vi "Start FFMpeg Process.vi"(8 "error in (no error)":errorcluster, 10 "Arguments":string, 11 "FFMPEG exe":path) -> (0 "error out":errorcluster, 3 "FFMpegProcess":T1)   [LabVIEW 2025]
uses:
  controls/FFMpegRef.ctl
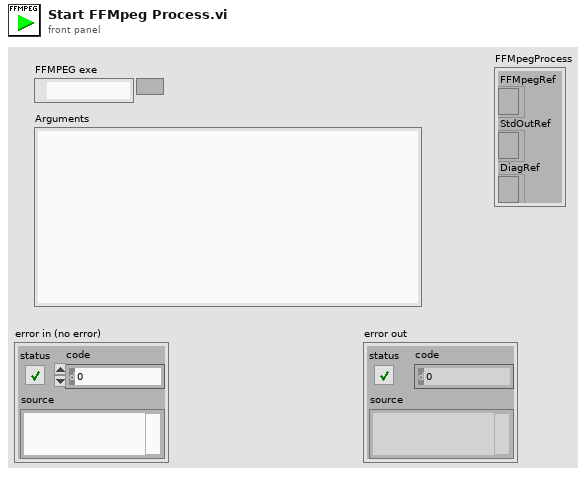
[diagram p1: front panel]
types:
  T1 = typedef "FFMpegRef.ctl" = cluster{"FFMpegRef":refnum<k24>, "StdOutRef":refnum<k24>, "DiagRef":refnum<k24>}
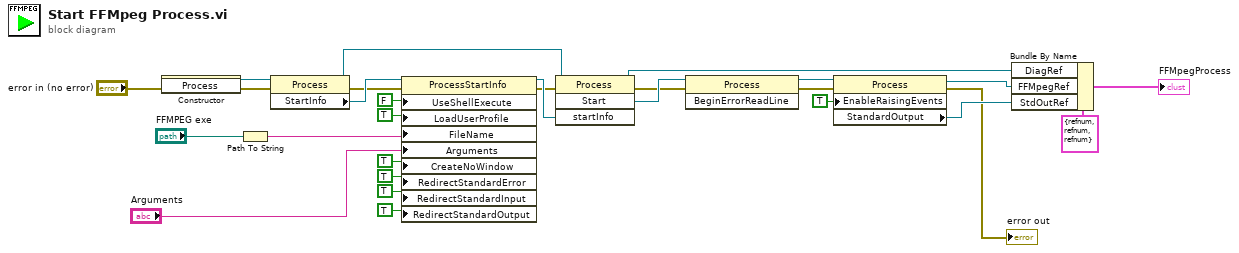
[diagram p0: block diagram]
diagram:
  n1 = constructor class="Process"(error in="error in (no error)") -> (reference out=w20:refnum<k24>, error out=w3:errorcluster)  [unwired: 2 in, 1 out]
  n2 = Path To String(path="FFMPEG exe") -> (string=w21:string)
  n3 = property class="Process"(reference=w20, error in=w3) -> (reference out=w22:refnum<k24>, error out=w8:errorcluster, "StartInfo"=w9:refnum<k24>)
  n4 = property class="ProcessStartInfo"(reference=w9, error in=w8, "UseShellExecute"=FALSE, "LoadUserProfile"=TRUE, "FileName"=w21, "Arguments"="Arguments", "CreateNoWindow"=TRUE, "RedirectStandardError"=TRUE ("RedirectStandardInput"), "RedirectStandardInput"=TRUE, "RedirectStandardOutput"=TRUE) -> (reference out=w5:refnum<k24>, error out=w4:errorcluster)
  n5 = invoke class="Process" method="Start"(reference=w22, error in=w4, "startInfo"=w5) -> (reference out=w26:refnum<k24>, error out=w13:errorcluster, "Start"=w19:refnum<k24>)  [unwired: 1 in, 1 out]
  n6 = invoke class="Process" method="BeginErrorReadLine"(reference=w19, error in=w13) -> (reference out=w12:refnum<k24>, error out=w14:errorcluster)  [unwired: 1 in, 1 out]
  n7 = property class="Process"(reference=w12, error in=w14, "EnableRaisingEvents"=TRUE) -> (reference out=w27:refnum<k24>, error out=→"error out":errorcluster, "StandardOutput"=w28:refnum<k24>)
  n8 = Bundle By Name(cluster=T1 {"FFMpegRef"=refnum, "StdOutRef"=refnum, "DiagRef"=refnum} ("FFMpegProcess"), "DiagRef"=w26, "FFMpegRef"=w27, "StdOutRef"=w28) -> (→"FFMpegProcess":T1)
